vi "Benchmarks.vi"() -> (0 "error out":errorcluster)   [LabVIEW 2012]
doc: "This code module is used for benchmarking the LabVIEW Adapter."
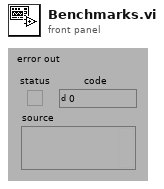
[diagram p1: front panel]
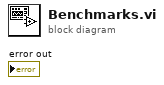
[diagram p0: block diagram]
diagram:
